vi "2-1.vi"() -> ()   [LabVIEW 2019, in "2.lvlib"]
uses:
  2.lvlib
  <vilib>/Utility/file.llb/Read Delimited Spreadsheet (string).vi
panel:
  out "XY Graph":cluster{i32[], i32[]}(graph)
  out "depth x distance":i32
  out "distance":i32
  out "depth":i32
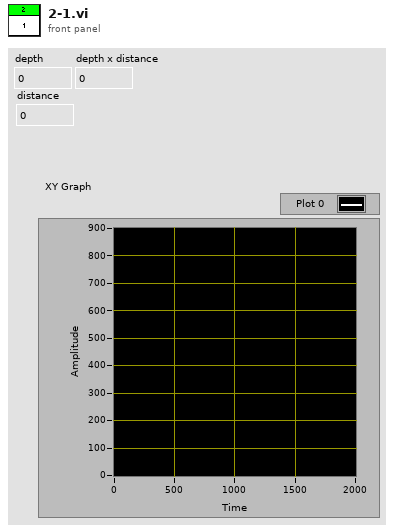
[diagram p1: front panel]
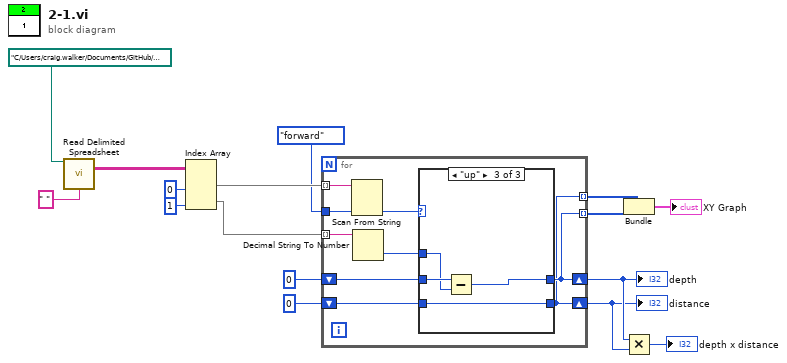
[diagram p0: block diagram]
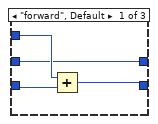
[diagram p2: hidden frame]
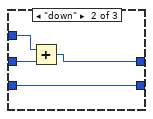
[diagram p3: hidden frame]
diagram:
  n1 = call-poly <vilib>:"Read Delimited Spreadsheet.vi"("file path (dialog if empty)"=path "C:/Users/craig.walker/Documents/GitHub/lv2019-Advent-of-Code-2021/2/input.txt", "delimiter (\\t)"=" " ("delimiter (\\t)")) -> ("all rows"=w16:string[][])  [unwired: 8 in, 5 out]
  n2 = Index Array(array=w16, index (col) #1=0 ("disabled index (col)"), index (col) #2=1 ("index (col)")) -> (element #1=w13:string[], element #2=w9:string[])  [unwired: 2 in]
  n3 = for {
    tunnel: w13 -> [w25] mode=indexing
    tunnel: enum16{"forward", "down", "up"}."forward" -> [w24]
    tunnel: w9 -> [w23] mode=indexing
    shift-right: [w18] -> w6
    shift-left: 0 -> [w21]
    shift-right: [w17] -> w5
    shift-left: 0 -> [w19]
    tunnel: [w18] -> w2 mode=indexing
    tunnel: [w17] -> w3 mode=indexing
    n4 = Scan From String(input string=w25, default 1=w24) -> (output 1=w22:enum16{"forward", "down", "up"})  [unwired: 3 in, 3 out]
    n5 = Decimal String To Number(string=w23) -> (number=w20:i32)  [unwired: 2 in, 1 out]
    n6 = case shown="\"up\"" w22 {
      tunnel: w21 -> [w27 w33 w37]
      tunnel: w20 -> [w28 w32 w36]
      tunnel: [w27 w31 w35] -> w18
      tunnel: w19 -> [w29 w30 w34]
      tunnel: [w26 w30 w34] -> w17
      frame "forward", Default {
        n7 = Add(x=w28, y=w29) -> (x+y=w26:i32)
      }
      frame "down" {
        n8 = Add(x=w32, y=w33) -> (x+y=w31:i32)
      }
      frame "up" {
        n9 = Subtract(x=w37, y=w36) -> (x-y=w35:i32)
      }
    }
  }
  "depth" <- w6
  "distance" <- w5
  n10 = Bundle(w3, w2) -> (→"XY Graph":cluster{i32[], i32[]})  [unwired: 1 in]
  n11 = Multiply(x=w6, y=w5) -> (x*y=→"depth x distance":i32)
